vi "RegisterLicense.vi"(8 "key":string, 9 "licensee":string, 11 "error in (no error)":errorcluster) -> (0 "status":string, 1 "state":i32(ring) items=["Invalid"=0, "Trial"=1, "ExtraTrial"=2, "Expired"=3, "MaintenanceNeeded"=4, "Licensed"=5, "None"=-1], 3 "error out":errorcluster)   [LabVIEW 2024, in "UnderAutomation.Fanuc.lvlib"]
uses:
  UnderAutomation.Fanuc.lvlib
  C:/Users/fg/Documents/Fanuc.vi/LabVIEW_2024/UnderAutomation.Fanuc/lib/UnderAutomation.Fanuc.dll
  lib/UnderAutomation.Fanuc.dll
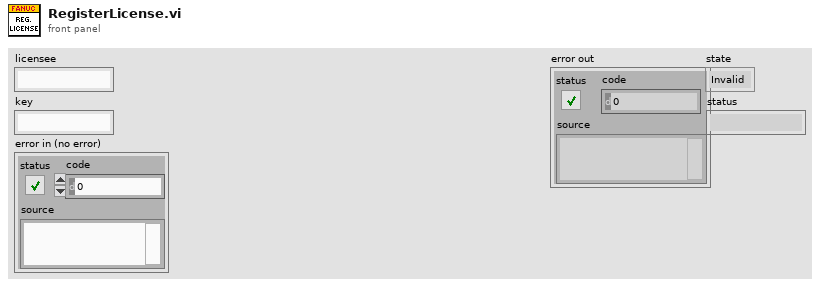
[diagram p1: front panel]
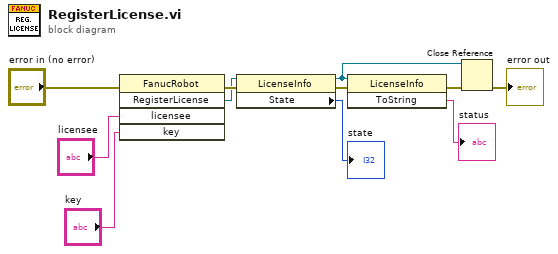
[diagram p0: block diagram]
diagram:
  n1 = invoke class="FanucRobot" method="RegisterLicense"(error in="error in (no error)", "licensee"="licensee", "key"="key") -> (error out=w6:errorcluster, "RegisterLicense"=w2:refnum<k24>)  [unwired: 2 in, 3 out]
  n2 = property class="LicenseInfo"(reference=w2, error in=w6) -> (reference out=w3:refnum<k24>, error out=w5:errorcluster, "State"=→"state":i32)
  n3 = invoke class="LicenseInfo" method="ToString"(reference=w3, error in=w5) -> (error out=w1:errorcluster, "ToString"=→"status":string)  [unwired: 1 in, 1 out]
  n4 = Close Reference(reference=w3, error in (no error)=w1) -> (error out=→"error out":errorcluster)
